vi "History Length.vi"(8 "Error In":errorcluster, 10 "History Length":u32, 11 "BNT_XtGraph in":refnum<class "BNT_XtGraph.lvclass">) -> (0 "Error Out":errorcluster, 3 "BNT_XtGraph out":refnum<class "BNT_XtGraph.lvclass">)   [LabVIEW 2019, in "BNT_XtGraph.lvlib" / "BNT_XtGraph.lvclass"]
doc: "Set history length, maximum samples per plot."
uses:
  BNT_XtGraph.lvclass
  BNT_XtGraph.lvclass/BNT_XtGraph.ctl
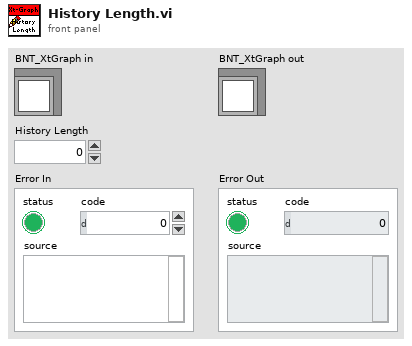
[diagram p1: front panel]
types:
  T1 = cluster{"X-t Value Pairs":cluster{"Time Stamp":timestamp, "Value":dbl}[]}[]
  T2 = cluster{"X-t Value Pairs":cluster{"Time Stamp":timestamp, "Value":dbl}[]}
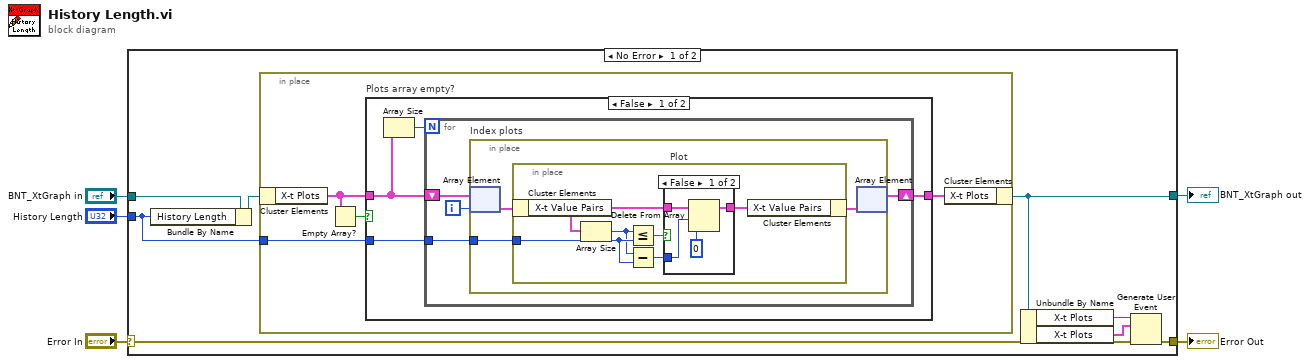
[diagram p0: block diagram]
diagram:
  n1 = case shown="No Error" "Error In" {
    selector: "Error In" -> [w11 w42]
    tunnel: [w12 w42] -> w3
    tunnel: [w13 w41] -> w2
    tunnel: "BNT_XtGraph in" -> [w9 w41]
    tunnel: "History Length" -> [w6 _]
    frame No Error {
      n2 = Bundle By Name(cluster=w9, "History Length"=w6) -> (w10:refnum<class "BNT_XtGraph.lvclass">)
      n3 = in-place {
        in-place-border: w6 -> [w14]
        n4 = in-place-cluster #1(w10) -> ("X-t Plots"=w15:T1)
        n5 = Empty Array?(array=w15) -> (empty?=w17:bool)
        n6 = case "Plots array empty?" shown="False" w17 {
          tunnel: [w20 w40] -> w16
          tunnel: w15 -> [w21 w40]
          tunnel: w14 -> [w19 _]
          frame False {
            n7 = Array Size(array=w21) -> (size(s)=w18:i32)
            n8 = for {
              N: w18 -> [_]
              shift-right: [w23] -> w20
              shift-left: w21 -> [w25]
              tunnel: w19 -> [w22]
              i -> [w24]
              n9 = in-place "Index plots" {
                in-place-border: w22 -> [w26]
                n10 = in-place-array #2(w25, w24) -> (w28:T2)
                n11 = in-place "Plot" {
                  in-place-border: w26 -> [w31]
                  n12 = in-place-cluster #3(w28) -> ("X-t Value Pairs"=w33:cluster{"Time Stamp":timestamp, "Value":dbl}[])
                  n13 = Array Size(array=w33) -> (size(s)=w30:i32)
                  n14 = Less Or Equal?(x=w30, y=w31) -> (x <= y?=w34:bool)
                  n15 = Subtract(x=w30, y=w31) -> (x-y=w29:u32)
                  n16 = case shown="False" w34 {
                    tunnel: w33 -> [w38 w39]
                    tunnel: [w37 w39] -> w32
                    tunnel: w29 -> [w35 _]
                    frame False {
                      n17 = Delete From Array(array=w38, length=w35, index=0) -> (array with subset deleted=w37:cluster{"Time Stamp":timestamp, "Value":dbl}[])  [unwired: 1 out]
                    }
                    frame True {
                    }
                  }
                  n18 = in-place-cluster #3("X-t Value Pairs"=w32) -> (w27:T2)
                }
                n19 = in-place-array #2(w27) -> (w23:T1)  [unwired: 1 out]
              }
            }
          }
          frame True {
          }
        }
        n20 = in-place-cluster #1("X-t Plots"=w16) -> (w13:refnum<class "BNT_XtGraph.lvclass">)
      }
      n21 = Unbundle By Name(w13) -> ("X-t Plots"=w8:refnum<user-event>, "X-t Plots"=w7:T1)
      n22 = Generate User Event(user event=w8, event data cluster=w7, error in=w11) -> (error out=w12:errorcluster)  [unwired: 1 in, 1 out]
    }
    frame Error {
    }
  }
  "BNT_XtGraph out" <- w2
  "Error Out" <- w3
